vi "refnums.vi"() -> ()   [LabVIEW 2019]
panel:
  out "Victor 3":string
  out "Victor 2":string
  out "Victor1":string
  out "Talon 3":string
  out "Talon 2":string
  out "Talon 1":string
  out "LED_2":string
  out "LED_1":string
  out "Wheel_4_Pot":string
  out "Wheel_3_Pot":string
  out "Wheel_2_Pot":string
  out "Wheel_1_Pot":string
  out "Wheel_4_Azimuth":string
  out "Wheel_3_Azimuth":string
  out "IMU_0":string
  out "Joystick_Driver":string
  out "Shifters":string
  out "Butterfly":string
  out "Compressor":string
  out "Wheel_2_Azimuth":string
  out "Wheel_1_Azimuth":string
  out "Wheel_4_Speed":string
  out "Wheel_3_Speed":string
  out "Wheel_2_Speed":string
  out "Wheel_1_Speed":string
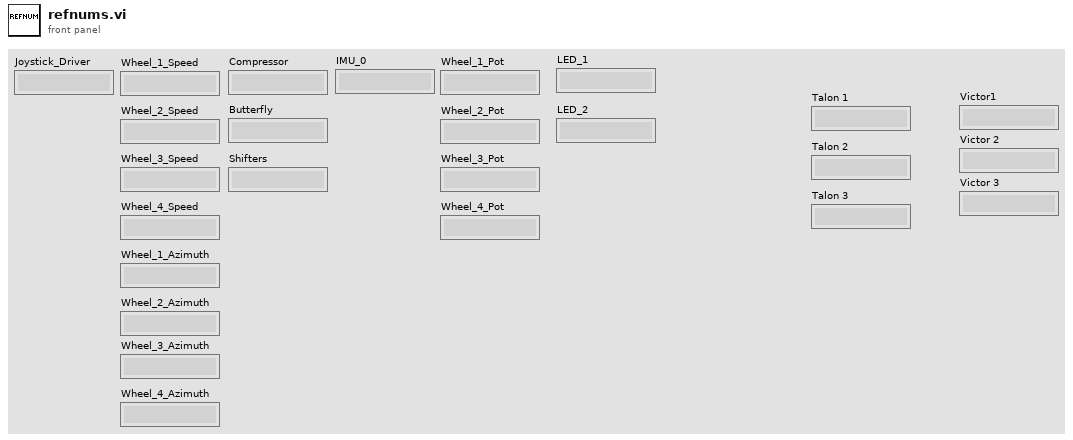
[diagram p1: front panel]
diagram:
